vi "Read Current Setpoint.vi"   [LabVIEW 2023, in "Current Control.lvclass"]
uses:
  Current Control.lvclass
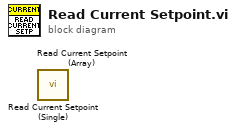
[diagram p0: block diagram]
diagram:
  n1 = call "Read Current Setpoint (Single).vi"() -> ()  [unwired: 8 in, 4 out]
  n2 = call "Read Current Setpoint (Array).vi"() -> ()  [unwired: 8 in, 4 out]
